vi "Plot Label StringToTime.vi"(2 "Time & Date Format String":string) -> (1 "UTC":i16, 4 "MDY":i16, 5 "Time Format":i16, 6 "AM/PM":i16, 7 "included seconds":i16, 8 "Date Format":i16, 9 "seconds precision":i16, 10 "Year Format":i16)   [LabVIEW 2017, in "2D Plot.lvclass"]
uses:
  <vilib>/Math Plots/2D Math Plots/2D Plot/2D Plot/2D Plot.lvclass
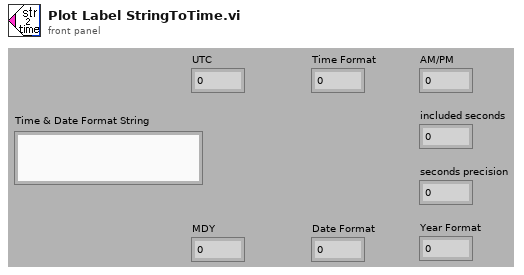
[diagram p1: front panel]
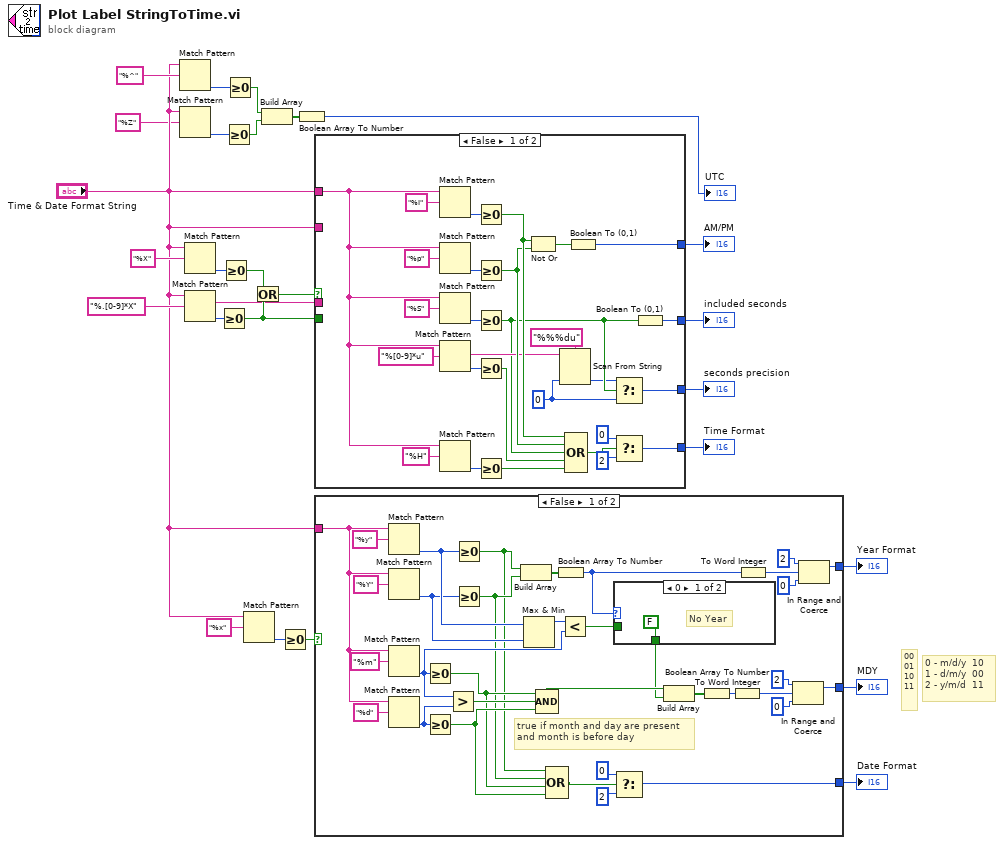
[diagram p0: block diagram]
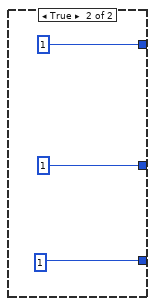
[diagram p3: hidden frame]
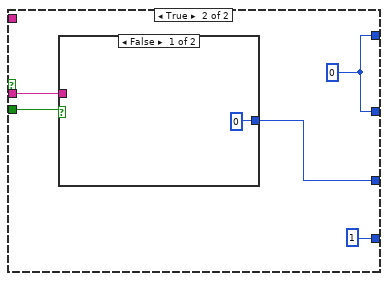
[diagram p4: hidden frame]
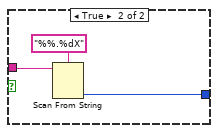
[diagram p5: hidden frame]
diagram:
  # "0 - m/d/y  10\n1 - d/m/y  00\n2 - y/m/d  11"
  # "00\n01\n10\n11"
  n1 = Match Pattern(string="Time & Date Format String", regular expression="%^") -> (offset past match=w8:i32)  [unwired: 4 out]
  n2 = Match Pattern(string="Time & Date Format String", regular expression="%Z") -> (offset past match=w5:i32)  [unwired: 4 out]
  n3 = Match Pattern(string="Time & Date Format String", regular expression="%X") -> (offset past match=w27:i32)  [unwired: 4 out]
  n4 = Match Pattern(string="Time & Date Format String", regular expression="%.[0-9]*X") -> (match substring=w10:string, offset past match=w14:i32)  [unwired: 3 out]
  n5 = Greater Or Equal To 0?(x=w14) -> (x >= 0?=w11:bool)
  n6 = Greater Or Equal To 0?(x=w27) -> (x >= 0?=w13:bool)
  n7 = Greater Or Equal To 0?(x=w5) -> (x >= 0?=w1:bool)
  n8 = Greater Or Equal To 0?(x=w8) -> (x >= 0?=w2:bool)
  n9 = Match Pattern(string="Time & Date Format String", regular expression="%x") -> (offset past match=w24:i32)  [unwired: 4 out]
  n10 = Or(x=w13, y=w11) -> (x .or. y?=w12:bool)
  n11 = Build Array(w2, w1) -> (w4:bool[])
  n12 = Greater Or Equal To 0?(x=w24) -> (x >= 0?=w23:bool)
  n13 = Boolean Array To Number(Boolean array=w4) -> (number=→"UTC":u32)
  n14 = case shown="False" w12 {
    tunnel: "Time & Date Format String" -> [w29 _]
    tunnel: [w41 i16 1] -> w22
    tunnel: [w39 w56] -> w21
    tunnel: [w38 w56] -> w20
    tunnel: [w33 w57] -> w19
    tunnel: "Time & Date Format String" -> [_ _]
    tunnel: w11 -> [_ w59]
    tunnel: w10 -> [_ w58]
    frame False {
      w32 = i16 0 ("f")
      n15 = Match Pattern(string=w29, regular expression="%I") -> (offset past match=w53:i32)  [unwired: 4 out]
      n16 = Match Pattern(string=w29, regular expression="%p") -> (offset past match=w52:i32)  [unwired: 4 out]
      n17 = Match Pattern(string=w29, regular expression="%S") -> (offset past match=w51:i32)  [unwired: 4 out]
      n18 = Match Pattern(string=w29, regular expression="%[0-9]*u") -> (match substring=w37:string, offset past match=w48:i32)  [unwired: 3 out]
      n19 = Match Pattern(string=w29, regular expression="%H") -> (offset past match=w31:i32)  [unwired: 4 out]
      n20 = Greater Or Equal To 0?(x=w53) -> (x >= 0?=w47:bool)
      n21 = Greater Or Equal To 0?(x=w52) -> (x >= 0?=w46:bool)
      n22 = Greater Or Equal To 0?(x=w51) -> (x >= 0?=w35:bool)
      n23 = Greater Or Equal To 0?(x=w48) -> (x >= 0?=w45:bool)
      n24 = Greater Or Equal To 0?(x=w31) -> (x >= 0?=w28:bool)
      n25 = Not Or(1:w46, 2:w47) -> (0:w40:bool)
      n26 = Scan From String(format string="%%%du", input string=w37, default 1=w32) -> (output 1=w34:i16)  [unwired: 2 in, 3 out]
      n27 = Compound Arithmetic op=OR(w47, w46, w35, w45, w28) -> (w44:bool)
      n28 = Boolean To (0,1)(Boolean=w40) -> (0, 1=w39:i16)
      n29 = Select(t=w34, s=w35, f=w32) -> (s? t:f=w33:i16)
      n30 = Select(t=i16 0, s=w44, f=i16 2) -> (s? t:f=w41:i16)
      n31 = Boolean To (0,1)(Boolean=w35) -> (0, 1=w38:i16)
    }
    frame True {
      w56 = i16 0
      n32 = case shown="False" w59 {
        tunnel: w58 -> [_ w64]
        tunnel: [i16 0 w62] -> w57
        frame False {
        }
        frame True {
          n33 = Scan From String(format string="%%.%dX", input string=w64) -> (output 1=w62:i32)  [unwired: 2 in, 4 out]
        }
      }
    }
  }
  "Time Format" <- w22
  "AM/PM" <- w21
  "included seconds" <- w20
  "seconds precision" <- w19
  n34 = case shown="False" w23 {
    tunnel: "Time & Date Format String" -> [w93 _]
    tunnel: [w90 i16 1 ("upper limit")] -> w18
    tunnel: [w76 i16 1 ("upper limit")] -> w16
    tunnel: [w68 i16 1 ("upper limit")] -> w17
    frame False {
      # "true if month and day are present\nand month is before day"
      n35 = Match Pattern(string=w93, regular expression="%y") -> (offset past match=w86:i32)  [unwired: 4 out]
      n36 = Match Pattern(string=w93, regular expression="%Y") -> (offset past match=w85:i32)  [unwired: 4 out]
      n37 = Match Pattern(string=w93, regular expression="%m") -> (offset past match=w83:i32)  [unwired: 4 out]
      n38 = Match Pattern(string=w93, regular expression="%d") -> (offset past match=w94:i32)  [unwired: 4 out]
      n39 = Greater Or Equal To 0?(x=w83) -> (x >= 0?=w74:bool)
      n40 = Greater Or Equal To 0?(x=w94) -> (x >= 0?=w75:bool)
      n41 = Greater?(x=w83, y=w94) -> (0:w87:bool)
      n42 = Greater Or Equal To 0?(x=w86) -> (x >= 0?=w72:bool)
      n43 = Greater Or Equal To 0?(x=w85) -> (x >= 0?=w73:bool)
      n44 = Build Array(w72, w73) -> (w92:bool[])
      n45 = Max & Min(x=w86, y=w85) -> (max(x,y)=w84:i32)  [unwired: 1 out]
      n46 = Compound Arithmetic op=AND(w74, w87, w75) -> (w77:bool)
      n47 = Compound Arithmetic op=OR(w72, w73, w74, w75) -> (w69:bool)
      n48 = Boolean Array To Number(Boolean array=w92) -> (number=w67:u32)
      n49 = Less?(x=w84, y=w83) -> (x < y?=w65:bool)
      n50 = case shown="0" w67 {
        tunnel: [FALSE w100] -> w66
        tunnel: w65 -> [_ w100]
        frame 0 {
          # "No Year"
        }
        frame Default {
          # "True if year is before month"
        }
      }
      n51 = Select(t=i16 0, s=w69, f=i16 2) -> (s? t:f=w68:i16)
      n52 = Build Array(w77, w66) -> (w78:bool[])
      n53 = Boolean Array To Number(Boolean array=w78) -> (number=w79:u32)
      n54 = To Word Integer(number=w79) -> (16bit integer=w80:i16)
      n55 = To Word Integer(number=w67) -> (16bit integer=w91:i16)
      n56 = In Range and Coerce(upper limit=i16 2, x=w80, lower limit=i16 0 ("upper limit")) -> (coerced(x)=w76:i16)  [unwired: 1 out]
      n57 = In Range and Coerce(upper limit=i16 2, x=w91, lower limit=i16 0 ("upper limit")) -> (coerced(x)=w90:i16)  [unwired: 1 out]
    }
    frame True {
    }
  }
  "Year Format" <- w18
  "Date Format" <- w17
  "MDY" <- w16
